vi "Remove Cashier.vi"(8 "error in (no error)":errorcluster, 10 "Cashier Index":i32, 11 "Coffee Shop in":refnum<class "Coffee Shop.lvclass">) -> (0 "error out":errorcluster, 3 "Coffee Shop out":refnum<class "Coffee Shop.lvclass">)   [LabVIEW 2023, in "Coffee Shop.lvlib" / "Coffee Shop.lvclass"]
doc: "Removes the Cashier stored at <b>Cashier Index</b>."
uses:
  Coffee Shop.lvclass
  Coffee Shop.lvclass/Coffee Shop.ctl
  Entity Types.ctl
  <vilib>/ActorFramework/Message Enqueuer/Message Enqueuer.lvclass/Message Enqueuer.ctl
  <vilib>/ActorFramework/Message Enqueuer/Enqueue.vi
  <vilib>/ActorFramework/Stop Msg/Stop Msg.lvclass
  c:/dev/_r/4/eng/lv-core/lvpostprocessingd/lv_mc_x86_64/dist_i386/vi.lib/ActorFramework/Message/Message.lvclass
  <vilib>/ActorFramework/Message Priority Queue/Priority Enqueue.vi
  Entity Table/Entity Table.lvclass
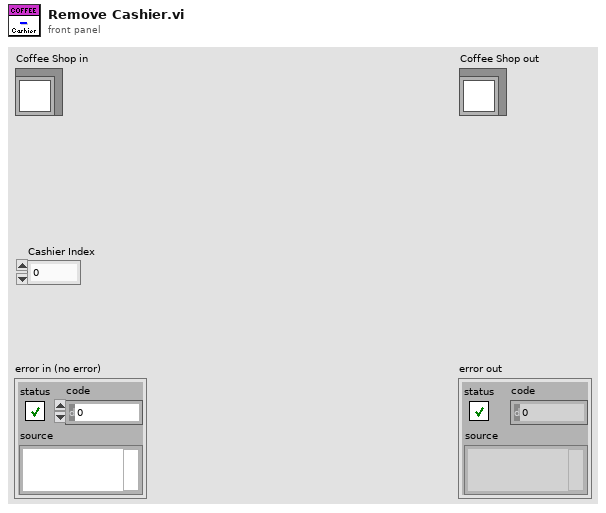
[diagram p1: front panel]
types:
  T1 = typedef "Coffee Shop.lvlib/Coffee Shop.lvclass/Entity Types.ctl" = enum16{"Customer", "Cashier", "Barista"}
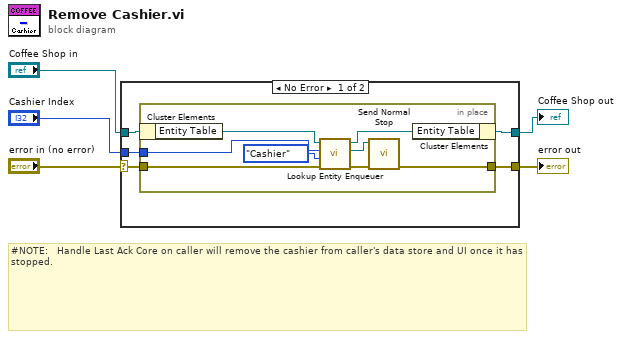
[diagram p0: block diagram]
diagram:
  # "#NOTE:   Handle Last Ack Core on caller will remove the cashier from caller's data store and UI once it has stopped."
  n1 = case shown="No Error" "error in (no error)" {
    selector: "error in (no error)" -> [w10 w20]
    tunnel: [w8 w20] -> w4
    tunnel: [w6 w19] -> w2
    tunnel: "Coffee Shop in" -> [w7 w19]
    tunnel: "Cashier Index" -> [w9 _]
    frame No Error {
      n2 = in-place "In Place Element Structure" {
        in-place-border: w10 -> [w18]
        in-place-border: w9 -> [w17]
        in-place-border: [w16] -> w8
        n3 = in-place-cluster #1 ("Unbundle / Bundle Elements")(w7) -> ("Entity Table"=w12:refnum<class "Entity Table.lvclass">)
        n4 = call "Lookup Entity Enqueuer.vi"("error in (no error)"=w18, "entity type"=Entity_Types."Cashier" ("Entity Type"), "entity index"=w17, "entity table in"=w12) -> ("error out"=w15:errorcluster, "entity"=w14:refnum<class "Message Enqueuer.lvclass">, "entity table out"=w11:refnum<class "Entity Table.lvclass">)  [unwired: 5 in]
        n5 = call <vilib>:"Send Normal Stop.vi"("error in (no error)"=w15, "Message Enqueuer"=w14) -> ("error out"=w16:errorcluster)  [unwired: 9 in]
        n6 = in-place-cluster #1 ("Unbundle / Bundle Elements")("Entity Table"=w11) -> (w6:refnum<class "Coffee Shop.lvclass">)
      }
    }
    frame Error {
    }
  }
  "error out" <- w4
  "Coffee Shop out" <- w2
